vi "Experiment header-Save_Load STATS section.vi"(4 "Logging queue element":T2={"Imaging Protocol"=enum."Live Imaging", "Number of Trials"=0, "Frame Size"=0, "# Averaged frames"=0, "Dwell time (us)"=0.1, "Index of Z-plane"=0, "Timelapse?"=FALSE, "Logging process is active"=FALSE, "Speed logging enabled"=FALSE, "tdms file ref"=refnum, "path"=path "", "Trial Number"=0, "Expected # points acquired"=FALSE, "Manually stopped"=FALSE, "Last trial"=FALSE, "Ch0 data"=[], "Ch1 data"=[], "Ref Data"=[], "Ref Frame Time"=[], "Image Time"=[], "Continuous Time"=[], "Ref X Length"=0, "Ref Y Length"=0, "# Ref Averaged frames"=0, "Ref Dwell time (us)"=0.0, "Points acquired"={"Ch0 last trial"=0, "Ch1 last trial"=0, "All trials"=0}, "HW Timings File"=refnum} {"Ref Dwell time (us)" format="%#.6g"; "Frame Size" items=["100X100"=100, "128X128"=128, "200X200"=200, "256X256"=256, "512X512"=512, "1024x1024"=1024, "2048x2048"=2048]; "Dwell time (us)" format="%#.6g"}, 8 "error in (no error)":errorcluster, 10 "Function":enum16{"Write", "Read"}(ring), 11 "Experiment folder path":path) -> (0 "error out":errorcluster, 1 "Read values":T1, 2 "Acquisition time unknown":bool)   [LabVIEW 2017]
uses:
  Typedefs/Logging queue element.ctl
  Typedefs/Imaging Protocols enum.ctl
  Typedefs/Frame Size.ctl
  Typedefs/Acquired points count.ctl
  Typedefs/Test header stats cluster.ctl
  Typedefs/Header file sections.ctl
  Typedefs/Header file interface module functions enum.ctl
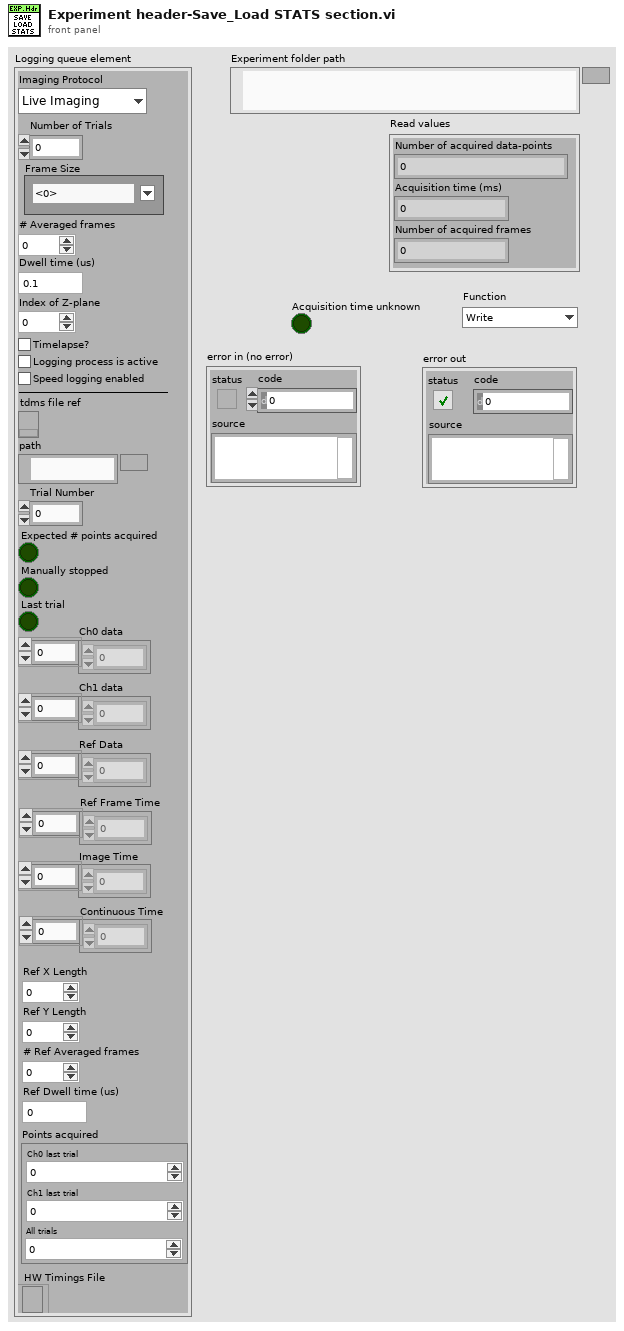
[diagram p1: front panel]
types:
  T1 = typedef "Test header stats cluster.ctl" = cluster{"Number of acquired data-points":dbl, "Acquisition time (ms)":dbl, "Number of acquired frames":dbl}
  T2 = typedef "Logging queue element.ctl" = cluster{"Imaging Protocol":T3, "Number of Trials":u16, "Frame Size":T4, "# Averaged frames":u16, "Dwell time (us)":dbl, "Index of Z-plane":i32, "Timelapse?":bool, "Logging process is active":bool, "Speed logging enabled":bool, "tdms file ref":refnum<k34>, "path":path, "Trial Number":i32, "Expected # points acquired":bool, "Manually stopped":bool, "Last trial":bool, "Ch0 data":u32[], "Ch1 data":u32[], "Ref Data":u32[], "Ref Frame Time":u64[], "Image Time":u64[], "Continuous Time":u64[], "Ref X Length":u16, "Ref Y Length":u16, "# Ref Averaged frames":u16, "Ref Dwell time (us)":dbl, "Points acquired":T5, "HW Timings File":refnum<file>}
  T3 = typedef "Imaging Protocols enum.ctl" = enum16{"AOL Z-Stack", "Motor Z Stack", "Functional Acquisition", "Single Plane Acquisition", "Volume Acquisition", "Live Imaging", "Live Plane Imaging", "Live Volume Imaging"}
  T4 = typedef "Frame Size.ctl" = u16
  T5 = typedef "Acquired points count.ctl" = cluster{"Ch0 last trial":u64, "Ch1 last trial":u64, "All trials":u64}
  T6 = typedef "Header file interface module functions enum.ctl" = enum16{"Load experiment header file", "Save experiment header file", "Clear stored values", "Read stored values", "Update specific value in memory", "Update values in memory"}
  T7 = typedef "Header file sections.ctl" = enum16{"ALL SECTIONS", "LOGIN", "GLOBAL PARAMETERS", "IMAGING MODES", "TIME SERIES", "MOTOR Z-STACK", "AOL Z-STACK", "FUNCTIONAL IMAGING", "VOLUME IMAGING", "MOVEMENT CORRECTION", "CALIBRATION", "STATISTICS", "BIOLOGY INFORMATION"}
  T8 = typedef "Fixed strings.ctl" = cluster{"ROI file name":string, "Normalised ROI file name":string, "Zplane Pockels values file name":string, "Functional data folder name":string, "Experiment Header file name":string, "Z-stack images folder name":string, "Groups setup rel. path":string, "Groups text file rel. path":string, "TDMS files folder name (F.img)":string, "TDMS files folder name (V.acq)":string, "TDMS files folder name (Pl.acq)":string, "Cycle rel times sequence file":string, "Dynamically called VIs folder name":string, "Time Series folder base name":string}
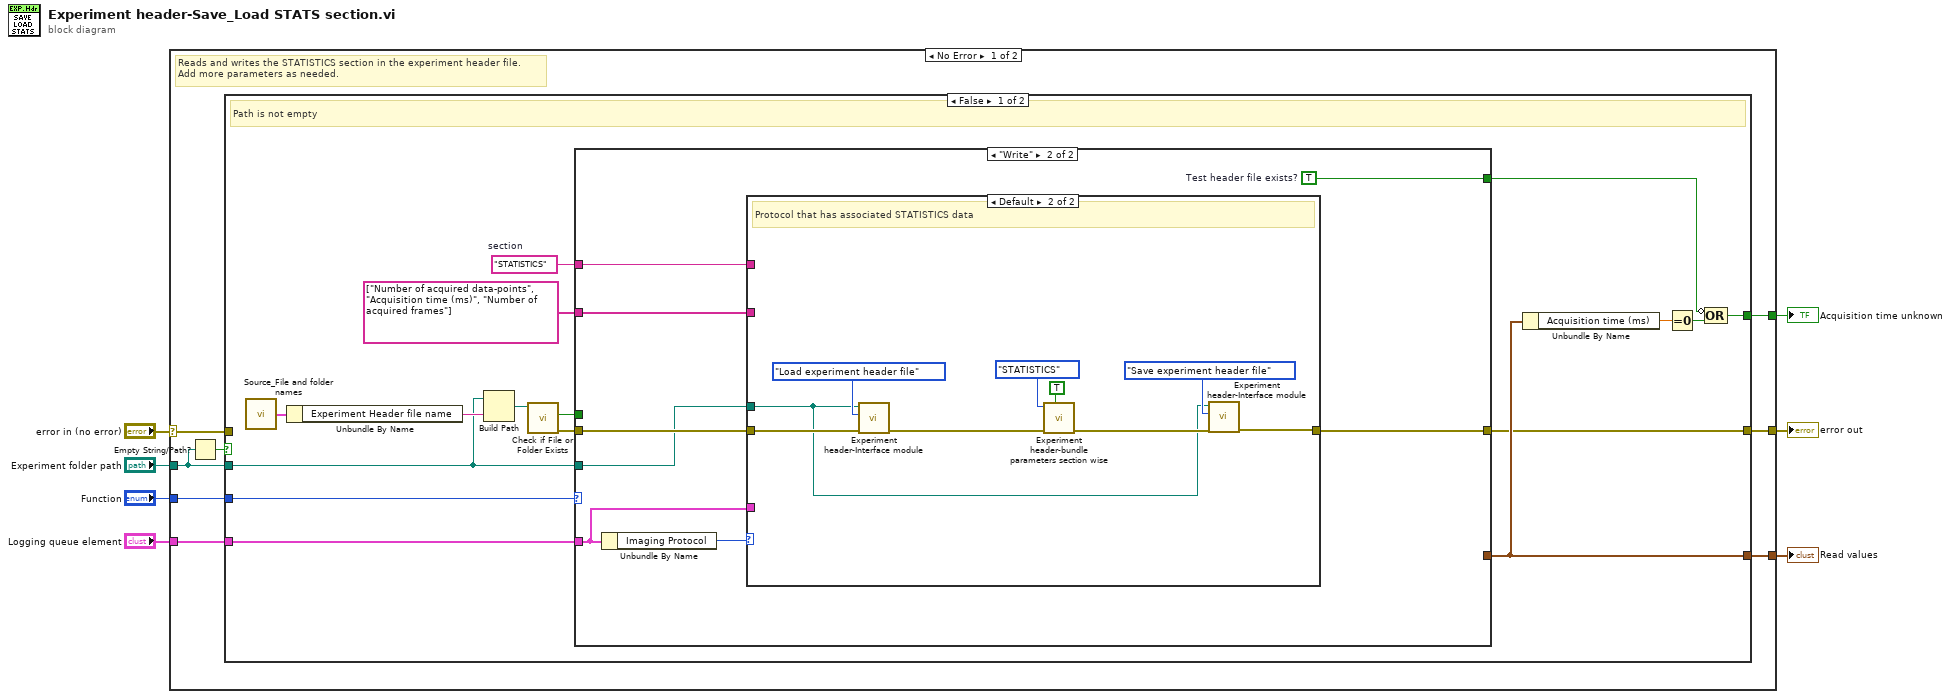
[diagram p0: block diagram]
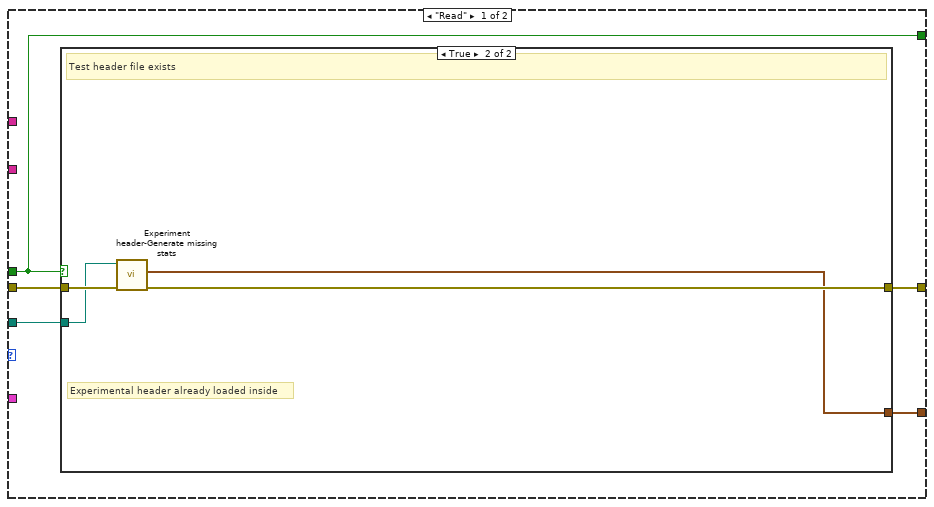
[diagram p2: hidden frame]
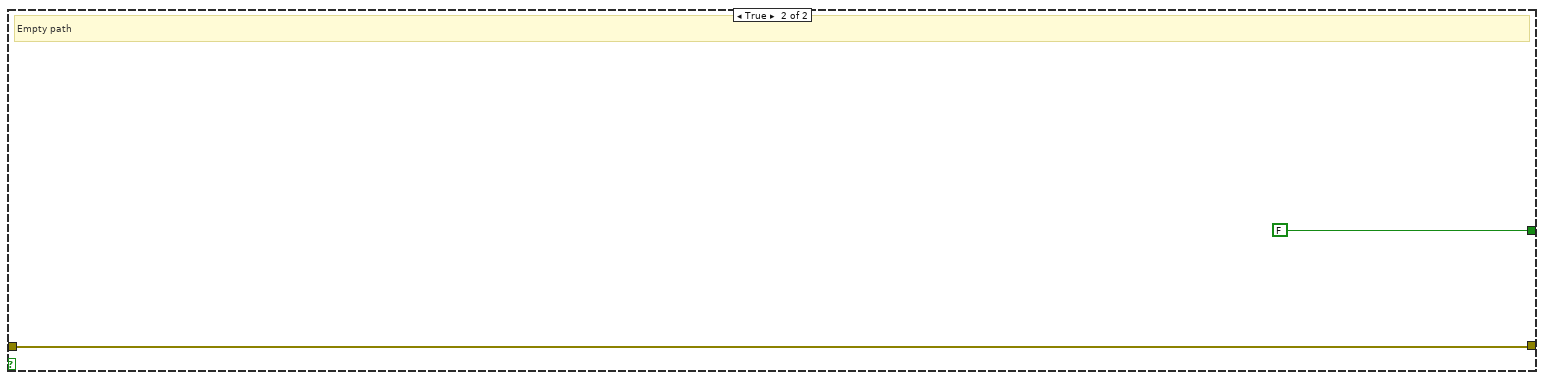
[diagram p5: hidden frame]
diagram:
  n1 = case shown="No Error" "error in (no error)" {
    selector: "error in (no error)" -> [w9 w62]
    tunnel: [w15 w62] -> w7
    tunnel: "Function" -> [w14 _]
    tunnel: "Experiment folder path" -> [w10 _]
    tunnel: "Logging queue element" -> [w13 _]
    tunnel: [w12 _] -> w3
    tunnel: [w8 _] -> w2
    frame No Error {
      # "Reads and writes the STATISTICS section in the experiment header file.\nAdd more parameters as needed."
      n2 = Empty String/Path?(string/path=w10) -> (empty?=w11:bool)
      n3 = case shown="False" w11 {
        tunnel: [w17 w61] -> w15
        tunnel: w14 -> [w20 _]
        tunnel: w10 -> [w21 _]
        tunnel: w13 -> [w22 _]
        tunnel: [w27 _] -> w12
        tunnel: w9 -> [_ w61]
        tunnel: [w24 FALSE ("File not found")] -> w8
        frame False {
          w23 = "STATISTICS"  # section
          # "Path is not empty"
          n4 = call "Source_File and folder names.vi"() -> ("Fixed strings"=w29:T8)  [unwired: 1 in]
          n5 = Unbundle By Name(w29) -> ("Experiment Header file name"=w30:string)
          n6 = Build Path(base path=w21, name or relative path=w30) -> (appended path=w28:path)
          n7 = call <vilib>:"Check if File or Folder Exists.vi"("path"=w28) -> ("error out"=w18:errorcluster, "file or folder exists?"=w19:bool)  [unwired: 8 in, 1 out]
          n8 = case shown="\"Write\"" w20 {
            tunnel: [w35 w43] -> w17
            tunnel: w18 -> [w36 w44]
            tunnel: w23 -> [_ w49]
            tunnel: string[] ["Number of acquired data-points", "Acquisition time (ms)", "Number of acquired frames"] -> [_ w48]
            tunnel: [w34 _] -> w27
            tunnel: w22 -> [_ w46]
            tunnel: w21 -> [w33 w42]
            tunnel: w19 -> [w32 _]
            tunnel: [w32 w45] -> w16
            frame "Read" {
              n9 = case shown="True" w32 {
                tunnel: w36 -> [w37 w41]
                tunnel: [w37 w40] -> w35
                tunnel: [_ w39] -> w34
                tunnel: w33 -> [_ w38]
                frame False {
                  # "Test header file doesnot exist"
                }
                frame True {
                  # "Experimental header already loaded inside"
                  # "Test header file exists"
                  n10 = call "Experiment header-Generate missing stats.vi"("error in (no error)"=w41, "Experiment folder path"=w38) -> ("error out"=w40:errorcluster, "STATS cluster"=w39:T1)  [unwired: 7 in, 1 out]
                }
              }
            }
            frame "Write" {
              w45 = TRUE  # Test header file exists?
              n11 = Unbundle By Name(w46) -> ("Imaging Protocol"=w47:T3)
              n12 = case shown="Default" w47 {
                tunnel: w49 -> [_ _]
                tunnel: [w50 w53] -> w43
                tunnel: w48 -> [_ _]
                tunnel: w46 -> [_ _]
                tunnel: w44 -> [w50 w56]
                tunnel: w42 -> [_ w51]
                frame "AOL Z-Stack", "Motor Z Stack" {
                  # "Protocols without associated STATISTICS data"
                }
                frame Default {
                  # "Protocol that has associated STATISTICS data"
                  n13 = call "Experiment header-Interface module.vi"("error in (no error)"=w56, "Function"=Header_file_interface_module_functions_enum."Load experiment header file", "Experiment data folder path"=w51) -> ("error out"=w55:errorcluster)  [unwired: 7 in, 1 out]
                  n14 = call "Experiment header-bundle parameters section wise.vi"("Update header\ninterface cluster ?"=TRUE ("Update header\ninterface cluster ?"), "error in (no error)"=w55, "Header file sections"=Header_file_sections."STATISTICS") -> ("error out"=w54:errorcluster)  [unwired: 7 in, 1 out]
                  n15 = call "Experiment header-Interface module.vi"("error in (no error)"=w54, "Function"=Header_file_interface_module_functions_enum."Save experiment header file", "Experiment data folder path"=w51) -> ("error out"=w53:errorcluster)  [unwired: 7 in, 1 out]
                }
              }
            }
          }
          n16 = Unbundle By Name(w27) -> ("Acquisition time (ms)"=w26:dbl)
          n17 = Equal To 0?(x=w26) -> (x = 0?=w25:bool)
          n18 = Compound Arithmetic op=OR(invert w16, w25) -> (w24:bool)
        }
        frame True {
          # "Empty path"
        }
      }
    }
    frame Error {
    }
  }
  "error out" <- w7
  "Read values" <- w3
  "Acquisition time unknown" <- w2
